vi "timeout.vi"(8 "error in (no error)":errorcluster, 11 "MonoHeartbeat in":refnum<class "MonoHeartbeat.lvclass">) -> (0 "error out":errorcluster, 2 "timeout?":bool, 3 "MonoHeartbeat out":refnum<class "MonoHeartbeat.lvclass">)   [LabVIEW 2016, in "MonoHeartbeat.lvclass"]
uses:
  MonoHeartbeat.lvclass
  MonoHeartbeat.lvclass/MonoHeartbeat.ctl
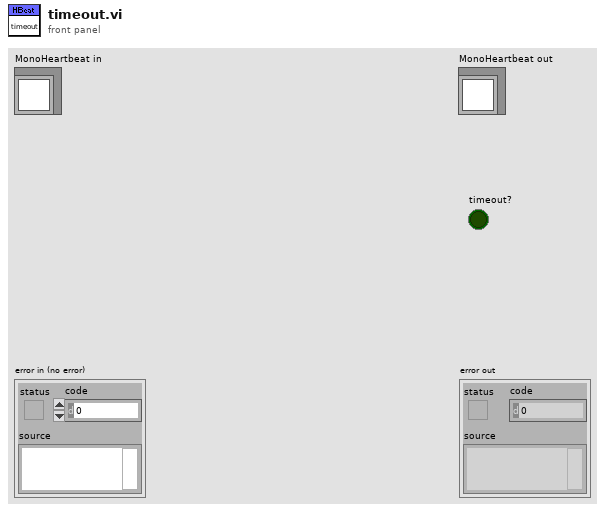
[diagram p1: front panel]
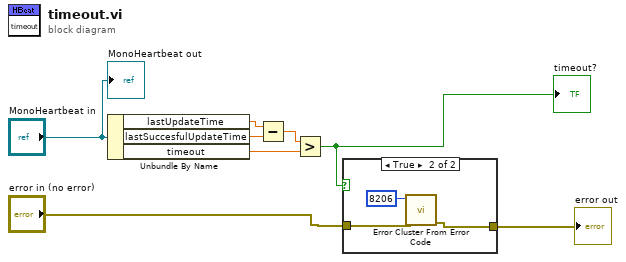
[diagram p0: block diagram]
diagram:
  n1 = Unbundle By Name("MonoHeartbeat in") -> ("lastUpdateTime"=w7:dbl, "lastSuccesfulUpdateTime"=w6:dbl, "timeout"=w4:dbl)
  n2 = Subtract(x=w7, y=w6) -> (x-y=w5:dbl)
  n3 = Greater?(x=w5, y=w4) -> (0:w3:bool)
  "timeout?" <- w3
  n4 = case shown="True" w3 {
    tunnel: "error in (no error)" -> [w9 w12]
    tunnel: [w9 w11] -> w1
    frame False {
    }
    frame True {
      n5 = call <vilib>:"Error Cluster From Error Code.vi"("error in (no error)"=w12, "error code (0)"=8206) -> ("error out"=w11:errorcluster)  [unwired: 7 in]
    }
  }
  "error out" <- w1
  "MonoHeartbeat out" <- "MonoHeartbeat in"
